vi "AlternatingLEDs.vi"() -> ()   [LabVIEW 2014]
uses:
  <vilib>/imath/engines/lvmath2/RunTimeEngine/Managers/WorkSpace/UID Generator.vi
  <vilib>/imath/engines/lvmath2/RunTimeEngine/BuiltInFunctions/mod/NIMS_mod_no_size_check.vi
  <instcachedir>/0/NIMS_mod_no_size_check_5393E3382FD241D281EEB71DA286C65B.lvgen/NIMS_mod_no_size_check_5393E3382FD241D281EEB71DA286C65B_008.vi
  <vilib>/imath/engines/lvmath2/RunTimeEngine/RunTimeType/NIMS_RunTimeType_From StrictType (excl LVString).vi
  <instcachedir>/0/NIMS_RunTimeType_From StrictType (excl LVString)_15A5391EEA9C4AACB9955AC755B83D29.lvgen/NIMS_RunTimeType_From StrictType (excl LVString)_15A5391EEA9C4AACB9955AC755B83D29_000.vi
  <vilib>/imath/engines/lvmath2/RunTimeEngine/LocalVariableDefStatement/MC_LocalVariableDefStatement_Display.vi
  <vilib>/imath/engines/lvmath2/RunTimeEngine/Managers/SymbolTable/Clear UID.vi
  <vilib>/imath/engines/lvmath2/RunTimeEngine/NodeEndStatement/NIMS_NodeEndStatement_Output.vi
  <instcachedir>/0/NIMS_NodeEndStatement_Output_53EC0D466D134D7ABD903AC30B43404B.lvgen/NIMS_NodeEndStatement_Output_53EC0D466D134D7ABD903AC30B43404B_011.vi
  <vilib>/imath/engines/lvmath2/RunTimeEngine/ErrorHandling/NIMS_Finalize Error.vi
  <vilib>/imath/engines/lvmath2/RunTimeEngine/Managers/SymbolTable/NIMS_WorkSpace.lvlib
panel:
  in  "End Loop":bool
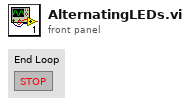
[diagram p1: front panel]
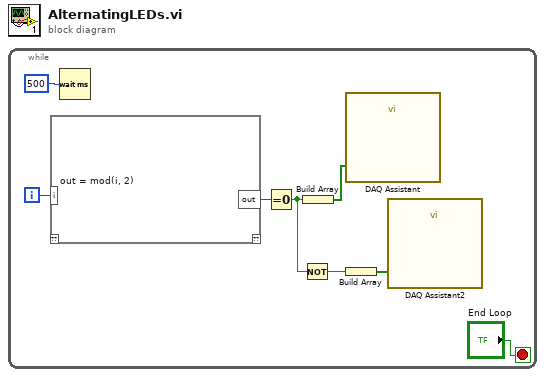
[diagram p0: block diagram]
diagram:
  n1 = while {
    i -> [w7]
    stop <- "End Loop" stop-if-true
    n2 = mathscript code="out = mod(i, 2)"("i"=w7) -> ("out"=w8:i32)  [unwired: 1 in, 1 out]
    n3 = Wait (ms)(milliseconds to wait=500) -> ()  [unwired: 1 out]
    n4 = Equal To 0?(x=w8) -> (x = 0?=w5:bool)
    n5 = Not(x=w5) -> (.not. x?=w4:bool)
    n6 = Build Array(w5) -> (w6:bool[])
    n7 = call "DAQ Assistant"("data"=w6) -> ()  [unwired: 17 in, 2 out]
    n8 = Build Array(w4) -> (w3:bool[])
    n9 = call "DAQ Assistant2"("data"=w3) -> ()  [unwired: 17 in, 2 out]
  }
